vi "SaveLayout.vi"(4 "Non-user layouts":cluster{"String":string, "Value":i32}[](array[cluster]), 6 "Layout Ring Refnum":refnum<vi>, 7 "Col Array Refnum":refnum<vi>, 8 "error in (no error)":errorcluster, 9 "ColLayout Array (empty)":T1[](array[typedef]), 10 "Local Layout ring":refnum<vi>, 11 "Trans LayoutInfo array in":T1[][](array[typedef])) -> (0 "error out":errorcluster, 1 "SaveError?":bool, 3 "Trans LayoutInfo array out":T1[][](array[typedef]))   [LabVIEW 2013]
uses:
  TypeDefs/ColumnLayout_UI.ctl
  ColumnVIs/Column/Column.lvclass
  TypeDefs/ColumnLayoutCluster.ctl
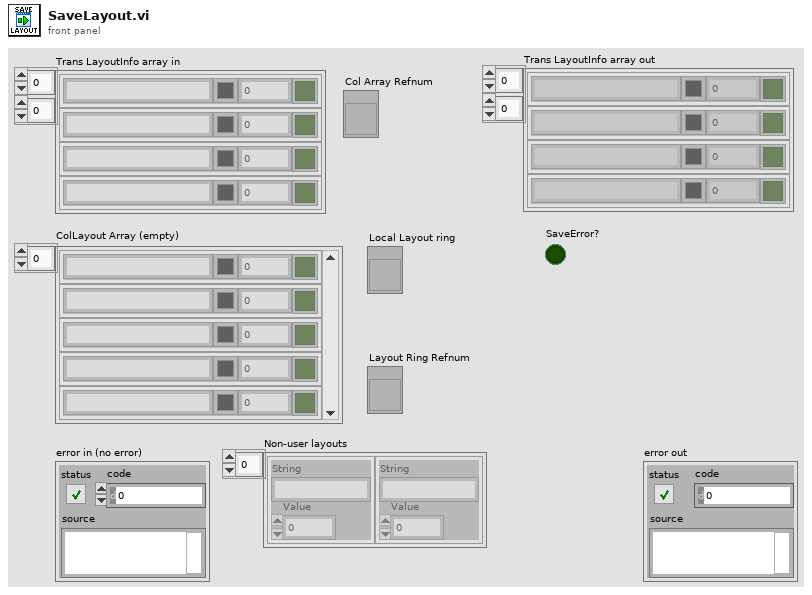
[diagram p1: front panel]
types:
  T1 = typedef "ColumnLayout_UI.ctl" = cluster{"Label":string, "Bgkd color":u32, "Width":u32, "Displayed?":bool}
  T2 = typedef "ColumnLayoutCluster.ctl" = cluster{"Label":string, "Color":u32, "Width":u32, "[disp?]":bool[]}
  T3 = typedef "LVStringsAndValuesArrayTypeDef_I32.ctl" = cluster{"String":string, "Value":i32}[]
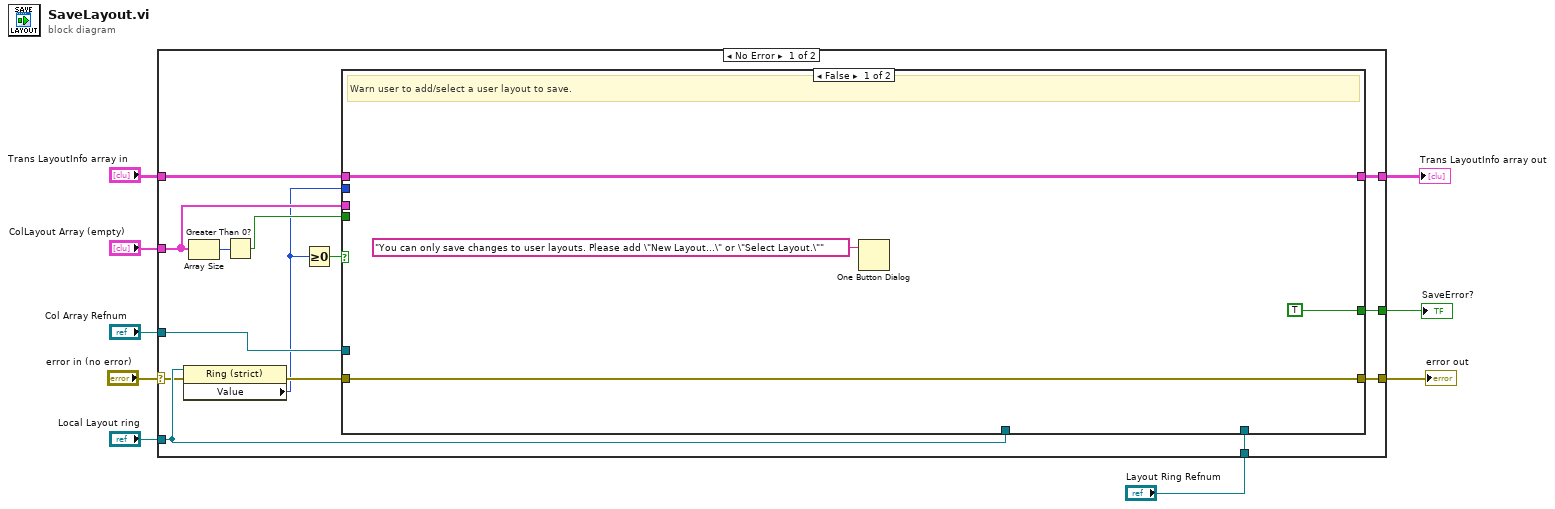
[diagram p0: block diagram]
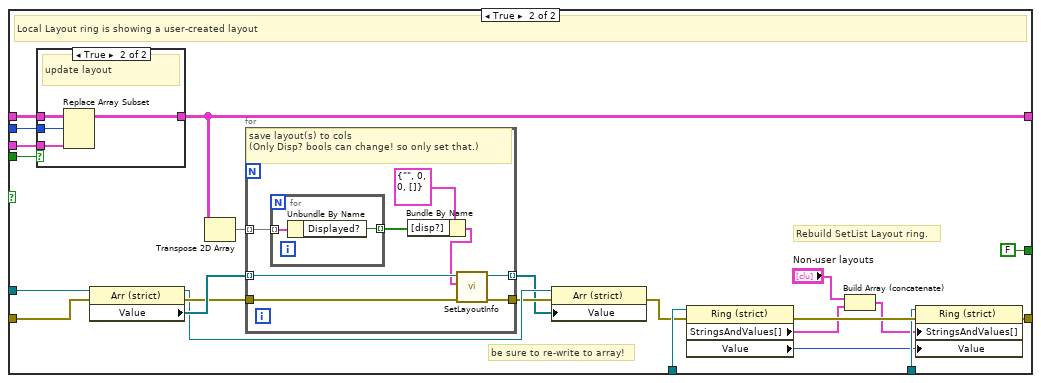
[diagram p2: hidden frame]
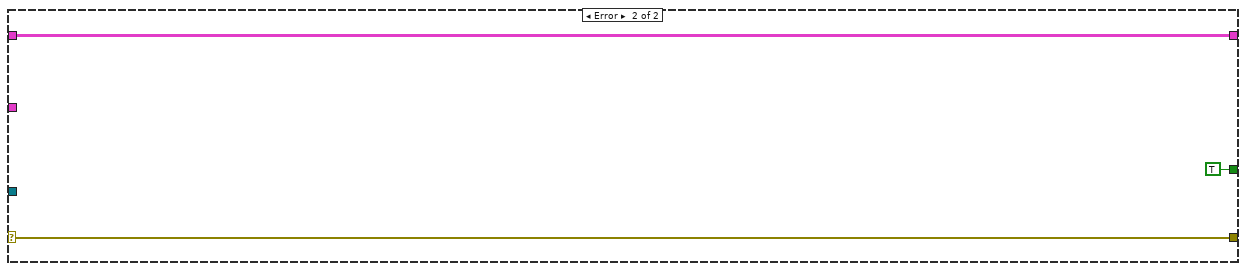
[diagram p4: hidden frame]
diagram:
  n1 = case shown="No Error" "error in (no error)" {
    selector: "error in (no error)" -> [w15 w68]
    tunnel: "Trans LayoutInfo array in" -> [w23 w67]
    tunnel: [w13 w67] -> w8
    tunnel: "ColLayout Array (empty)" -> [w21 _]
    tunnel: "Col Array Refnum" -> [w22 _]
    tunnel: [w18 w68] -> w4
    tunnel: "Layout Ring Refnum" -> [w17 _]
    tunnel: "Local Layout ring" -> [w16 _]
    tunnel: [w10 TRUE] -> w1
    frame No Error {
      n2 = property class="Ring (strict)"(reference=w16, error in=w15) -> (error out=w14:errorcluster, "Value"=w11:i32)  [unwired: 1 out]
      n3 = Array Size(array=w21) -> (size(s)=w20:i32)
      n4 = Greater Than 0?(x=w20) -> (x > 0?=w19:bool)
      n5 = Greater Or Equal To 0?(x=w11) -> (x >= 0?=w12:bool)
      n6 = case shown="False" w12 {
        tunnel: w23 -> [w27 w50]
        tunnel: w22 -> [_ w49]
        tunnel: w21 -> [_ w46]
        tunnel: w19 -> [_ w45]
        tunnel: [w26 w43] -> w18
        tunnel: w17 -> [_ w42]
        tunnel: w16 -> [_ w41]
        tunnel: w14 -> [w26 w40]
        tunnel: w11 -> [_ w39]
        tunnel: [w27 w38] -> w13
        tunnel: [TRUE FALSE] -> w10
        frame False {
          # "Warn user to add/select a user layout to save."
          n7 = One Button Dialog(message="You can only save changes to user layouts. Please add \"New Layout...\" or \"Select Layout.\"") -> ()  [unwired: 1 in, 1 out]
        }
        frame True {
          # "be sure to re-write to array!"
          # "Rebuild SetList Layout ring."
          # "Local Layout ring is showing a user-created layout"
          n8 = case shown="True" w45 {
            tunnel: w39 -> [_ w52]
            tunnel: w50 -> [w51 w55]
            tunnel: [w51 w54] -> w38
            tunnel: w46 -> [_ w53]
            frame False {
              # "no layout to update"
            }
            frame True {
              # "update layout"
              n9 = Replace Array Subset "Replace Array Subset"(array=w55, new element=w53, index (row)=w52) -> (w54:T1[][])  [unwired: 1 in]
            }
          }
          n10 = property class="Arr (strict)"(reference=w49, error in=w40) -> (reference out=w36:refnum<vi>, error out=w47:errorcluster, "Value"=w48:refnum<class "Column.lvclass">[])
          n11 = Transpose 2D Array(2D array=w38) -> (transposed array=w37:T1[][])
          n12 = for {
            tunnel: w48 -> [w63] mode=indexing
            tunnel: w37 -> [w59] mode=indexing
            tunnel: w47 -> [w62]
            tunnel: [w61] -> w35
            tunnel: [w60] -> w34 mode=indexing
            # "save layout(s) to cols\n(Only Disp? bools can change! so only set that.)"
            n13 = for {
              tunnel: w59 -> [w65] mode=indexing
              tunnel: [w64] -> w57 mode=indexing
              n14 = Unbundle By Name(w65) -> ("Displayed?"=w64:bool)
            }
            n15 = Bundle By Name(cluster=T2 {"Label"="", "Color"=0, "Width"=0, "[disp?]"=[]} ("Layout cluster"), "[disp?]"=w57) -> (w56:T2)
            n16 = call "SetLayoutInfo.vi"("error in (no error)"=w62, "Layout cluster"=w56, "Column in"=w63) -> ("error out"=w61:errorcluster, "Column out"=w60:refnum<class "Column.lvclass">)  [unwired: 7 in]
          }
          n17 = property class="Arr (strict)"(reference=w36, error in=w35, "Value"=w34) -> (error out=w33:errorcluster)  [unwired: 1 out]
          n18 = property on="Property Node" class="Ring (strict)"(reference=w41, error in=w33) -> (error out=w44:errorcluster, "StringsAndValues[]"=w30:T3, "Value"=w32:i32)  [unwired: 1 out]
          n19 = Build Array (concatenate)("Non-user layouts", w30) -> (w29:T3)
          n20 = property class="Ring (strict)"(reference=w42, error in=w44, "StringsAndValues[]"=w29, "Value"=w32) -> (error out=w43:errorcluster)  [unwired: 1 out]
        }
      }
    }
    frame Error {
    }
  }
  "error out" <- w4
  "Trans LayoutInfo array out" <- w8
  "SaveError?" <- w1
